vi "OpenY16DeviceByXML.vi"(2 "error in (no error)":errorcluster, 3 "Filename":string, 4 "ICImagingControl":refnum<k7>) -> (0 "error out":errorcluster, 1 "ICImagingControl 2":refnum<k7>)   [LabVIEW 2020]
doc: "This VI is for handling Y16 sink (pixelformat) only.\nOpen a camera using a previously created XML file. Create the XML with the DeviceXMLGenerator.exe in tne samples\\DeviceXMLGenerator directory.The OverlayBitmap is disabled."
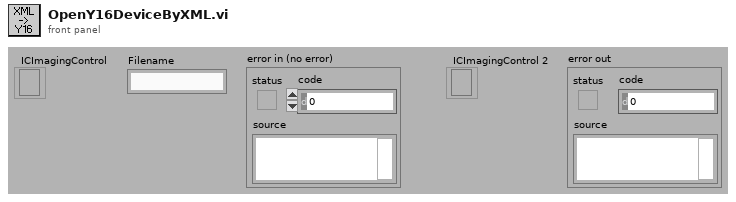
[diagram p1: front panel]
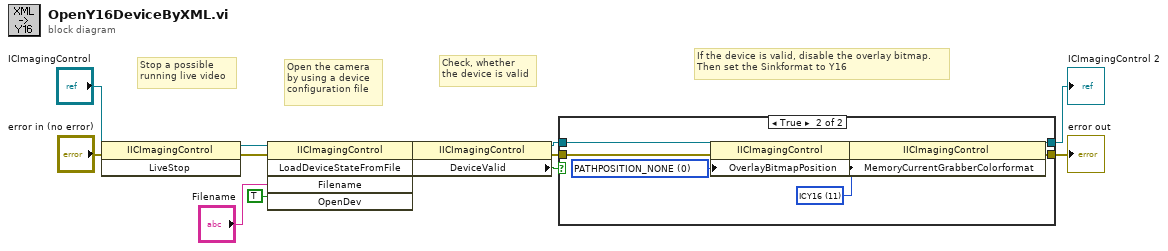
[diagram p0: block diagram]
diagram:
  # "If the device is valid, disable the overlay bitmap.\nThen set the Sinkformat to Y16"
  # "Check, whether\nthe device is valid"
  # "Open the camera\nby using a device \nconfiguration file"
  # "Stop a possible\nrunning live video"
  n1 = invoke class="IICImagingControl" method="LiveStop"(reference="ICImagingControl", error in="error in (no error)") -> (reference out=w11:refnum<k7>, error out=w12:errorcluster)  [unwired: 1 in, 1 out]
  n2 = invoke class="IICImagingControl" method="LoadDeviceStateFromFile"(reference=w11, error in=w12, "Filename"="Filename", "OpenDev"=TRUE) -> (reference out=w2:refnum<k7>, error out=w3:errorcluster)  [unwired: 1 in, 3 out]
  n3 = property class="IICImagingControl"(reference=w2, error in=w3) -> (reference out=w5:refnum<k7>, error out=w6:errorcluster, "DeviceValid"=w4:bool)
  n4 = case shown="True" w4 {
    tunnel: w5 -> [w15 w22]
    tunnel: [w15 w19] -> w7
    tunnel: w6 -> [w14 w18]
    tunnel: [w14 w16] -> w8
    frame False {
    }
    frame True {
      w20 = 11 items=["ICRGB32"=1, "ICRGB24"=2, "ICRGB565"=3, "ICRGB555"=4, "ICY8"=5, "ICUYVY"=6, "ICY800"=7, "ICYGB1"=8, "ICYGB0"=9, "ICBY8"=10, "ICY16"=11] ("MemoryCurrentGrabberColorformat")
      w23 = 0 items=["PATHPOSITION_NONE"=0, "PATHPOSITION_DEVICE"=1, "PATHPOSITION_SINK"=2, "PATHPOSITION_DISPLAY"=4] ("OverlayBitmapPosition")
      n5 = property class="IICImagingControl"(reference=w22, error in=w18, "OverlayBitmapPosition"=w23) -> (reference out=w21:refnum<k7>, error out=w17:errorcluster)
      n6 = property class="IICImagingControl"(reference=w21, error in=w17, "MemoryCurrentGrabberColorformat"=w20) -> (reference out=w19:refnum<k7>, error out=w16:errorcluster)
    }
  }
  "error out" <- w8
  "ICImagingControl 2" <- w7
